vi "read test.vi"() -> ()   [LabVIEW 2019]
uses:
  <vilib>/WPC Systems Ltd/GECO Driver/Lib/GECOBase/GECO_Driver Class/GECO_SlotName.ctl
  <vilib>/WPC Systems Ltd/GECO Driver/GECODriver/GECO_Initialize_RT/Initialize VIs/Initialize_GECOUnoRT_4HX.vi
  <vilib>/WPC Systems Ltd/GECO Driver/Lib/GECOBase/GECO_Driver Class/GECO_Driver.lvclass
panel:
  out "program period":u32
  in  "stop":bool
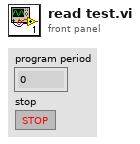
[diagram p1: front panel]
types:
  T1 = typedef "GECO_Driver.lvclass/GECO_SlotName.ctl" = enum16{"C1", "C2", "C3", "C4"}
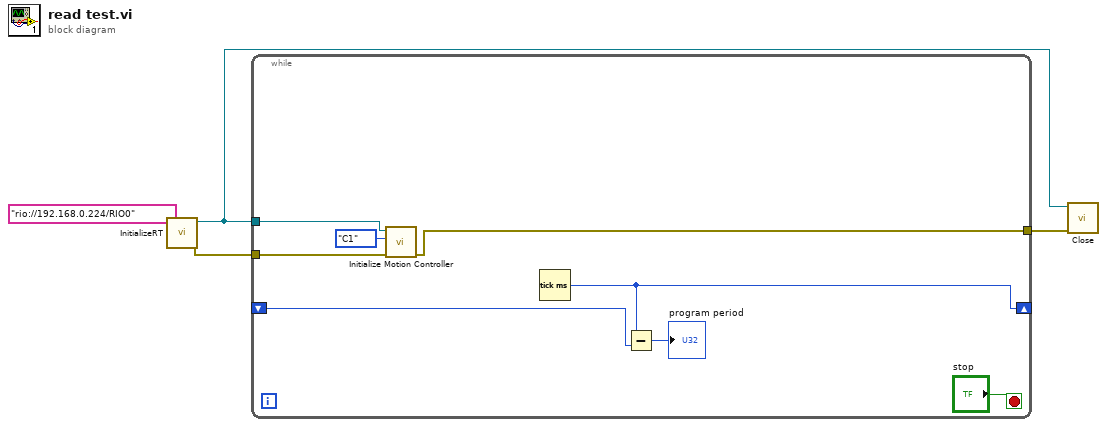
[diagram p0: block diagram]
diagram:
  n1 = call-poly <vilib>:"InitializeRT.vi"("resource name"=tag "rio://192.168.0.224/RIO0") -> ("error out"=w3:errorcluster, "GECO_Driver out"=w2:refnum<class "GECO_Driver.lvclass">)  [unwired: 9 in]
  n2 = while {
    shift-right: [w10] -> _
    shift-left: _ -> [w11]
    tunnel: w3 -> [w8]
    tunnel: w2 -> [w7]
    tunnel: [w5] -> w1
    stop <- "stop" stop-if-true
    n3 = call <vilib>:"Initialize Motion Controller.vi"("error in (no error)"=w8, "Slot"=GECO_SlotName."C1", "GECO_Driver in"=w7) -> ("error out"=w5:errorcluster)  [unwired: 7 in, 1 out]
    n4 = Tick Count (ms)() -> (millisecond timer value=w10:u32)
    n5 = Subtract(x=w10, y=w11) -> (x-y=→"program period":u32)
  }
  n6 = call <vilib>:"Close.vi"("error in (no error)"=w1, "GECO_Driver in"=w2) -> ()  [unwired: 9 in, 1 out]
